vi "SS_FPGA_Drop1_all_in_v1.vi"() -> ()   [LabVIEW 2016]
uses:
  <vilib>/rvi/Emulation/niFpgaGetClockAttributes.vi
  <vilib>/rvi/Emulation/niFpgaSctlEmulationGetInTimedLoop.vi
  <vilib>/rvi/Emulation/niFpgaEmulationReportErrorSimple.vi
  <vilib>/rvi/Emulation/niFpgaCriticalErrorInLSC.vi
  <vilib>/rvi/Emulation/niFpgaProcessEmulError.vi
  <vilib>/rvi/eio/common/nirviEmuTemplateMethod_errors.vi
  <vilib>/eio/EIONode/EIONode.xnode
panel:
  in  "Scan Rate (mSec) Loop 3":u32 caption="Count(mSec)"
  out "Actual Duration (ms) 3":u32
  in  "Scan Rate (mSec) Loop 2":u32 caption="Count(mSec)"
  out "Actual Duration (ms) 2":u32
  in  "Set Pump Interlock":bool
  out "Raw Data out Mod 3":fxp<+/-,24,-4>[](array[numeric]) format="%.27g"
  out "Raw Data out Mod 2":fxp<+/-,24,-4>[](array[numeric]) format="%.27g"
  in  "Scan Rate (mSec) Loop 1":u32 caption="Count(mSec)"
  out "Raw Data out Mod 1":fxp<+/-,24,-4>[](array[numeric]) format="%.27g"
  out "Number of Loop 1 Samples":i32
  out "Actual Duration (ms)":u32
  in  "Set Flow Interlock":bool
  in  "Start Acquisition":bool
  # "SS Source Body Flow\n\nSS Source Body Temperature\n\nSS Grid 1 Flow\n\nSS Grid 1 Temperature\n\nSS Grid 2 Flow\n\nSS Grid 2 Temperature\n\nSS Grid 3 Flow\n\nSS Grid 3 Temperature\n\nSS Grid 4/1st Stage Neutraliser Flow\n\nSS Grid 4/1st Stage Neutraliser Temperature\n\nSS 2nd Stage Neutraliser Flow\n\nSS 2nd Stage Neutraliser Temperature\n\nSS PINI Backplate Flow\n\nSS PINI Backplate Temperature\n\nSS Duct Scraper Flow\n\nSS Duct Scraper Temperature"
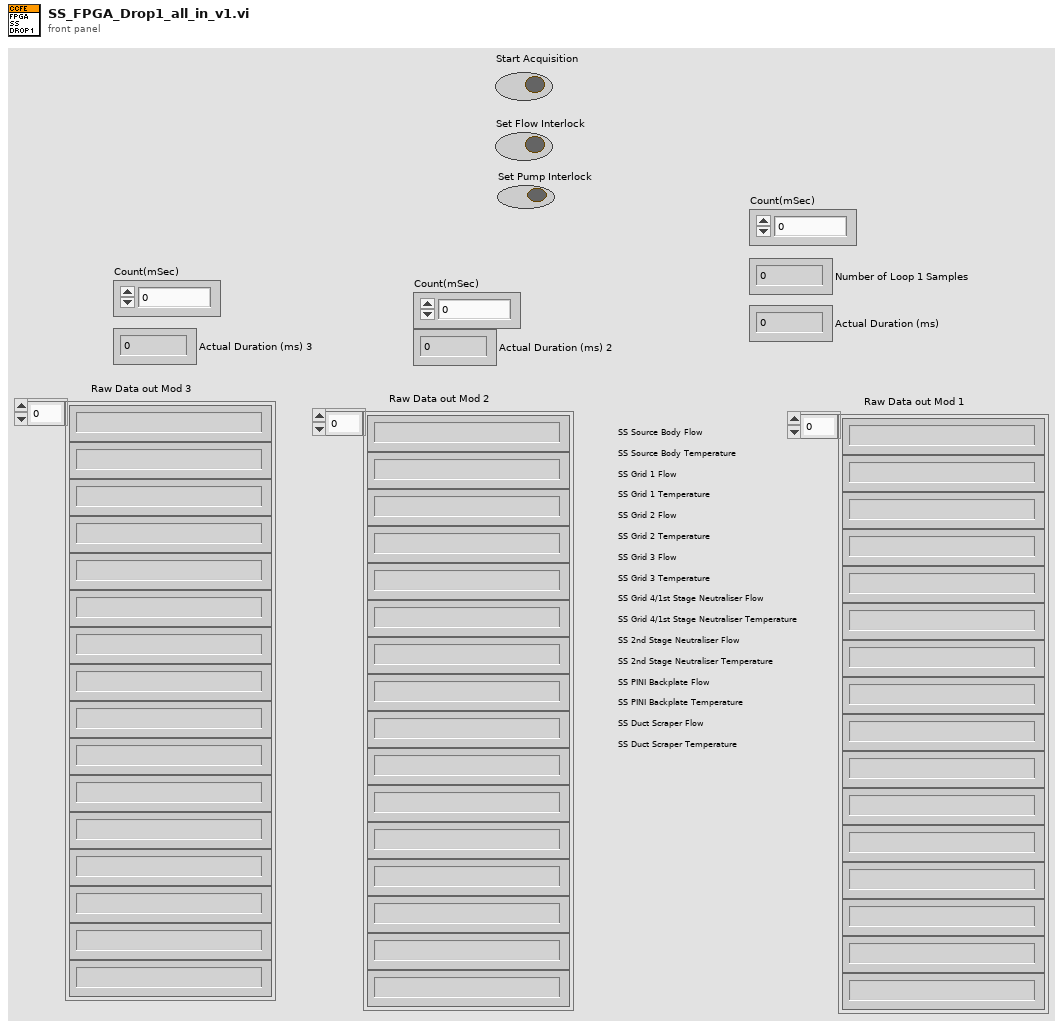
[diagram p1: front panel]
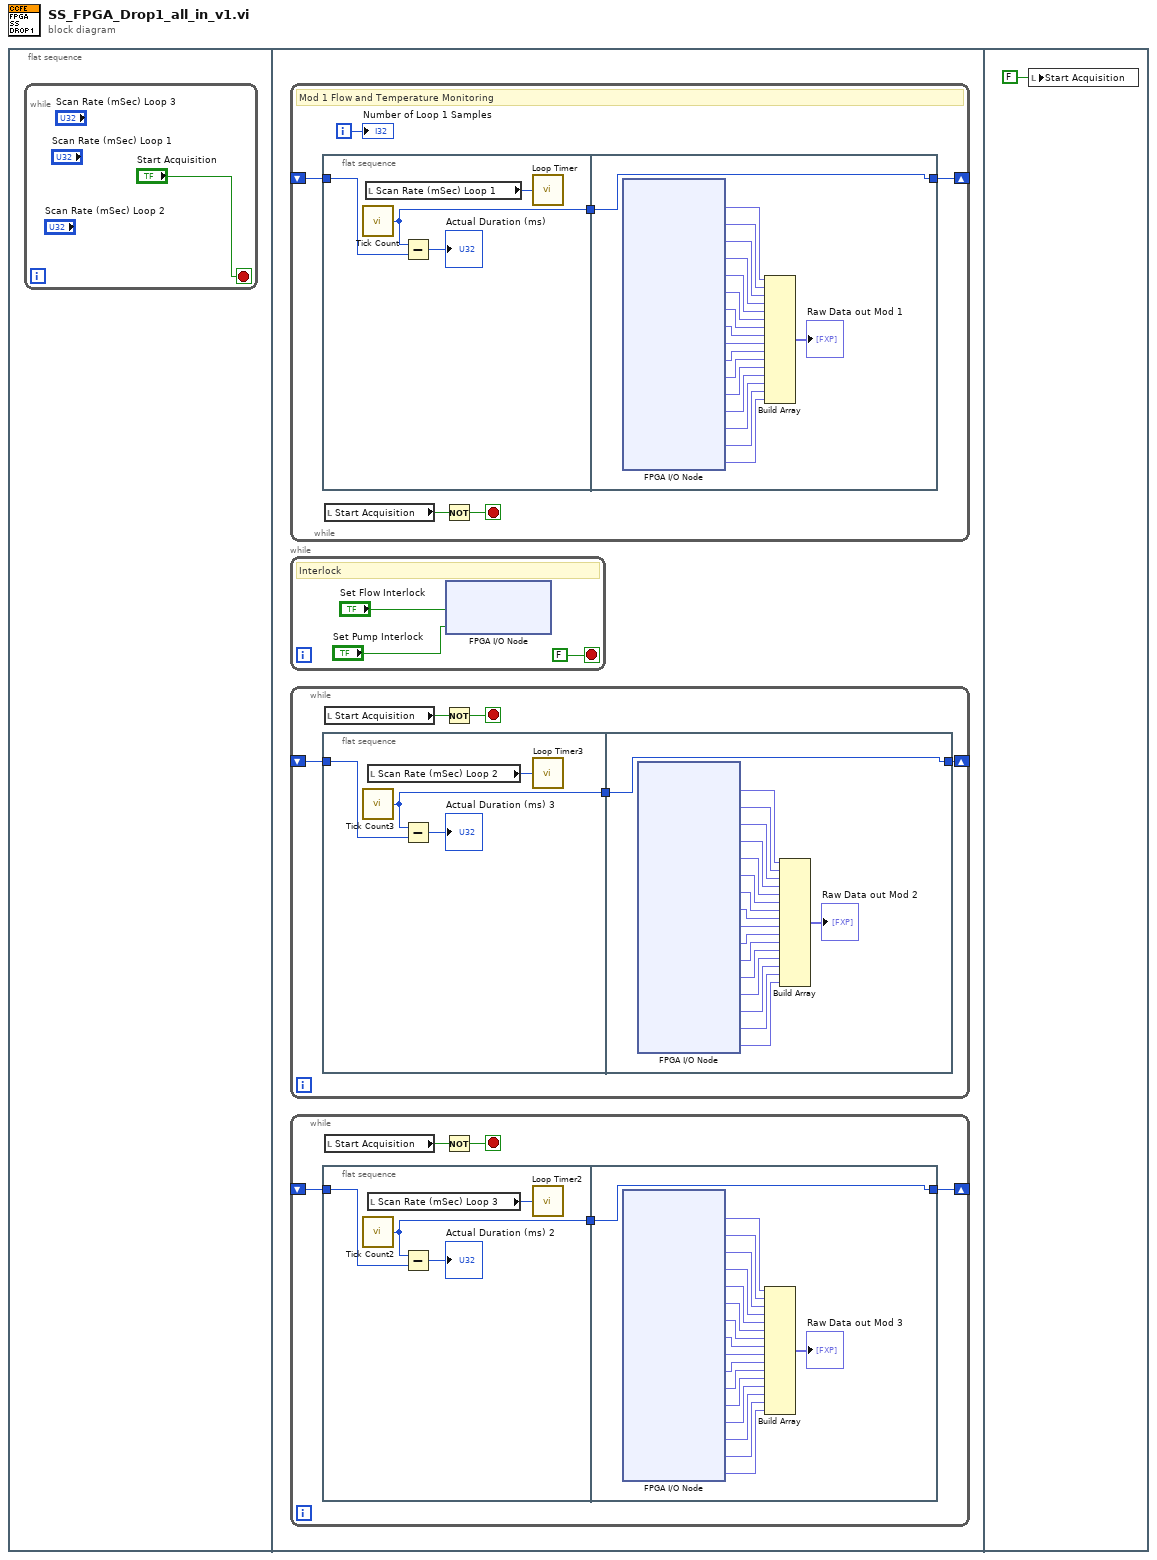
[diagram p0: block diagram]
diagram:
  n1 = flat-sequence {
    frame #0 {
      n2 = while {
        stop <- "Start Acquisition" stop-if-true
      }
    }
    frame #1 {
      n3 = while {
        shift-right: [w63] -> _
        shift-left: _ -> [w61]
        i -> [w64]
        stop <- w60 stop-if-true
        # "Mod 1 Flow and Temperature Monitoring"
        n4 = flat-sequence {
          tunnel: [w65] -> w62
          tunnel: w61 -> [w66]
          tunnel: [w69] -> w63
          tunnel: w62 -> [w69]
          frame #0 {
            n5 = call "Tick Count"() -> ("Tick Count(mSec)"=w65:u32)
            n6 = local read "Scan Rate (mSec) Loop 1"() -> (w68:u32)
            n7 = Subtract(x=w65, y=w66) -> (x-y=→"Actual Duration (ms)":u32)
            n8 = call "Loop Timer"("Count(mSec)"=w68) -> ()  [unwired: 1 out]
          }
          frame #1 {
            n9 = xnode "FPGA I/O Node"() -> ("Mod1/AI0"=w86:fxp<+/-,24,-4>, "Mod1/AI1"=w85:fxp<+/-,24,-4>, "Mod1/AI2"=w84:fxp<+/-,24,-4>, "Mod1/AI3"=w83:fxp<+/-,24,-4>, "Mod1/AI4"=w82:fxp<+/-,24,-4>, "Mod1/AI5"=w81:fxp<+/-,24,-4>, "Mod1/AI6"=w80:fxp<+/-,24,-4>, "Mod1/AI7"=w79:fxp<+/-,24,-4>, "Mod1/AI8"=w78:fxp<+/-,24,-4>, "Mod1/AI9"=w77:fxp<+/-,24,-4>, "Mod1/AI10"=w76:fxp<+/-,24,-4>, "Mod1/AI11"=w75:fxp<+/-,24,-4>, "Mod1/AI12"=w74:fxp<+/-,24,-4>, "Mod1/AI13"=w73:fxp<+/-,24,-4>, "Mod1/AI14"=w72:fxp<+/-,24,-4>, "Mod1/AI15"=w71:fxp<+/-,24,-4>)  [unwired: 16 in, 16 out]
            n10 = Build Array(w86, w85, w84, w83, w82, w81, w80, w79, w78, w77, w76, w75, w74, w73, w72, w71) -> (→"Raw Data out Mod 1":fxp<+/-,24,-4>[])
          }
        }
        n11 = local read "Start Acquisition"() -> (w59:bool)
        n12 = Not(x=w59) -> (.not. x?=w60:bool)
        "Number of Loop 1 Samples" <- w64
      }
      n13 = while {
        stop <- FALSE stop-if-true
        # "Interlock"
        n14 = xnode "FPGA I/O Node"("Mod6/DIO0"="Set Flow Interlock", "Mod6/DIO1"="Set Pump Interlock") -> ()  [unwired: 2 in, 2 out]
      }
      n15 = while {
        shift-right: [w4] -> _
        shift-left: _ -> [w2]
        stop <- w6 stop-if-true
        n16 = flat-sequence {
          tunnel: [w8] -> w3
          tunnel: w2 -> [w7]
          tunnel: [w11] -> w4
          tunnel: w3 -> [w11]
          frame #0 {
            n17 = call "Tick Count3"() -> ("Tick Count(mSec)"=w8:u32)
            n18 = local read "Scan Rate (mSec) Loop 2"() -> (w9:u32)
            n19 = Subtract(x=w8, y=w7) -> (x-y=→"Actual Duration (ms) 3":u32)
            n20 = call "Loop Timer3"("Count(mSec)"=w9) -> ()  [unwired: 1 out]
          }
          frame #1 {
            n21 = xnode "FPGA I/O Node"() -> ("Mod2/AI0"=w28:fxp<+/-,24,-4>, "Mod2/AI1"=w27:fxp<+/-,24,-4>, "Mod2/AI2"=w26:fxp<+/-,24,-4>, "Mod2/AI3"=w25:fxp<+/-,24,-4>, "Mod2/AI4"=w24:fxp<+/-,24,-4>, "Mod2/AI5"=w23:fxp<+/-,24,-4>, "Mod2/AI6"=w22:fxp<+/-,24,-4>, "Mod2/AI7"=w21:fxp<+/-,24,-4>, "Mod2/AI8"=w20:fxp<+/-,24,-4>, "Mod2/AI9"=w19:fxp<+/-,24,-4>, "Mod2/AI10"=w18:fxp<+/-,24,-4>, "Mod2/AI11"=w17:fxp<+/-,24,-4>, "Mod2/AI12"=w16:fxp<+/-,24,-4>, "Mod2/AI13"=w15:fxp<+/-,24,-4>, "Mod2/AI14"=w14:fxp<+/-,24,-4>, "Mod2/AI15"=w13:fxp<+/-,24,-4>)  [unwired: 16 in, 16 out]
            n22 = Build Array(w28, w27, w26, w25, w24, w23, w22, w21, w20, w19, w18, w17, w16, w15, w14, w13) -> (→"Raw Data out Mod 2":fxp<+/-,24,-4>[])
          }
        }
        n23 = local read "Start Acquisition"() -> (w5:bool)
        n24 = Not(x=w5) -> (.not. x?=w6:bool)
      }
      n25 = while {
        shift-right: [w34] -> _
        shift-left: _ -> [w32]
        stop <- w36 stop-if-true
        n26 = flat-sequence {
          tunnel: [w38] -> w33
          tunnel: w32 -> [w37]
          tunnel: [w41] -> w34
          tunnel: w33 -> [w41]
          frame #0 {
            n27 = call "Tick Count2"() -> ("Tick Count(mSec)"=w38:u32)
            n28 = local read "Scan Rate (mSec) Loop 3"() -> (w40:u32)
            n29 = Subtract(x=w38, y=w37) -> (x-y=→"Actual Duration (ms) 2":u32)
            n30 = call "Loop Timer2"("Count(mSec)"=w40) -> ()  [unwired: 1 out]
          }
          frame #1 {
            n31 = xnode "FPGA I/O Node"() -> ("Mod3/AI0"=w58:fxp<+/-,24,-4>, "Mod3/AI1"=w57:fxp<+/-,24,-4>, "Mod3/AI2"=w56:fxp<+/-,24,-4>, "Mod3/AI3"=w55:fxp<+/-,24,-4>, "Mod3/AI4"=w54:fxp<+/-,24,-4>, "Mod3/AI5"=w53:fxp<+/-,24,-4>, "Mod3/AI6"=w52:fxp<+/-,24,-4>, "Mod3/AI7"=w51:fxp<+/-,24,-4>, "Mod3/AI8"=w50:fxp<+/-,24,-4>, "Mod3/AI9"=w49:fxp<+/-,24,-4>, "Mod3/AI10"=w48:fxp<+/-,24,-4>, "Mod3/AI11"=w47:fxp<+/-,24,-4>, "Mod3/AI12"=w46:fxp<+/-,24,-4>, "Mod3/AI13"=w45:fxp<+/-,24,-4>, "Mod3/AI14"=w44:fxp<+/-,24,-4>, "Mod3/AI15"=w43:fxp<+/-,24,-4>)  [unwired: 16 in, 16 out]
            n32 = Build Array(w58, w57, w56, w55, w54, w53, w52, w51, w50, w49, w48, w47, w46, w45, w44, w43) -> (→"Raw Data out Mod 3":fxp<+/-,24,-4>[])
          }
        }
        n33 = local read "Start Acquisition"() -> (w35:bool)
        n34 = Not(x=w35) -> (.not. x?=w36:bool)
      }
    }
    frame #2 {
      n35 = local write "Start Acquisition"(FALSE ("Start Acquisition")) -> ()
    }
  }
